vi "Set Properties from Initial.vi"(8 "error in(no error)":errorcluster, 10 "Initial Value":variant, 11 "Properties in":variant) -> (0 "error out":errorcluster, 2 "type":T1, 3 "Properties out":variant)   [LabVIEW 2018, in "Tag Engine.lvlib" / "Tag.lvclass"]
uses:
  Tag.lvclass
  <vilib>/Utility/Data Type/Type Definitions/Data Type.ctl
  <vilib>/Utility/Data Type/NI_Data Type.lvlib
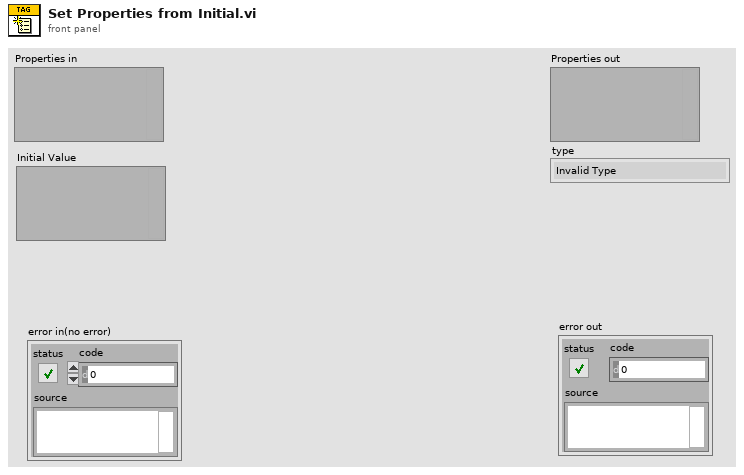
[diagram p1: front panel]
types:
  T1 = typedef "NI_Data Type.lvlib/Data Type.ctl" = enum8{"Invalid Type", "Void", "I8", "I16", "I32", "I64", "U8", "U16", "U32", "U64", "Single Float", "Double Float", "Extended Float", "Single Complex", "Double Complex", "Extended Complex", "Enum U8", "Enum U16", "Enum U32", "Enum U64", "Single Float With Unit", "Double Float With Unit", "Extended Float With Unit", "Single Complex with Unit", "Double Complex with Unit", "Extended Complex with Unit", "Boolean", "String", "Path", "Picture", "Tag", "Array", "Cluster", "Variant", "LV Variant", "Waveform", "Timestamp", "Digital Waveform", "Digital Data", "ExpressData", "Refnum", "External Data", "VI", "Poly VI", "LabVIEW Class Instance", "Fixed Point"}
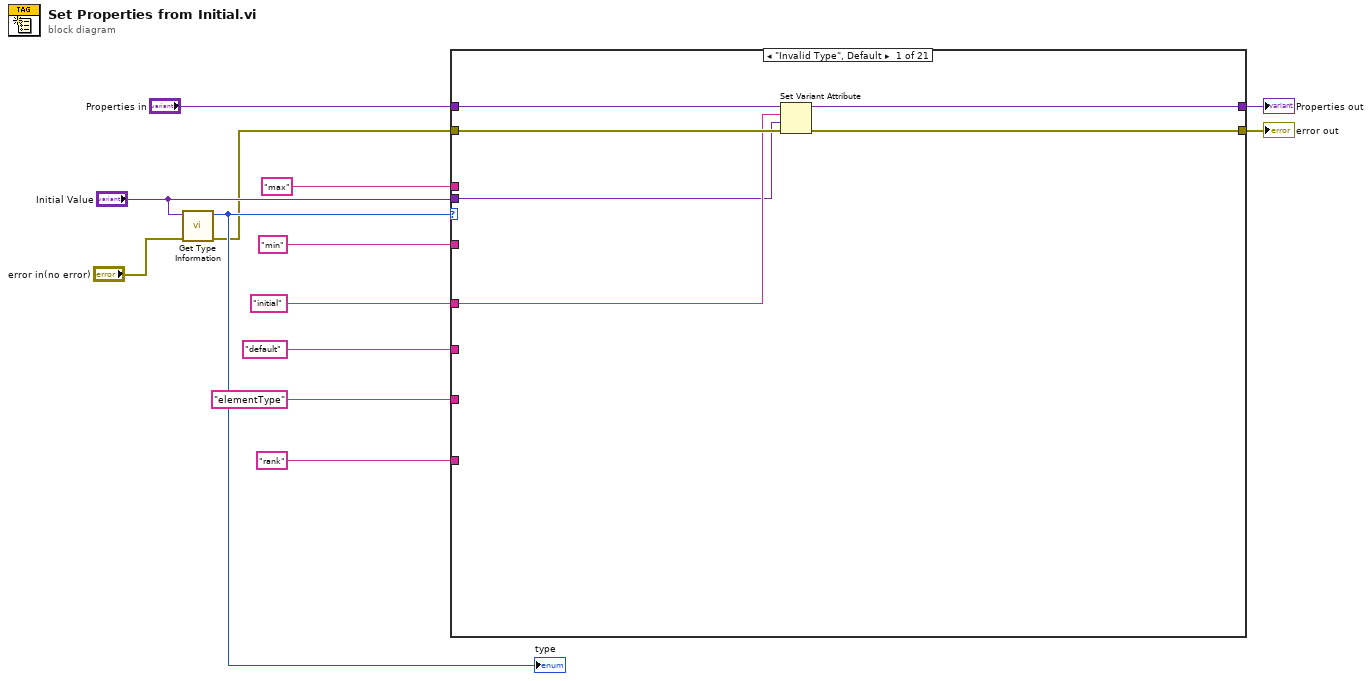
[diagram p0: block diagram]
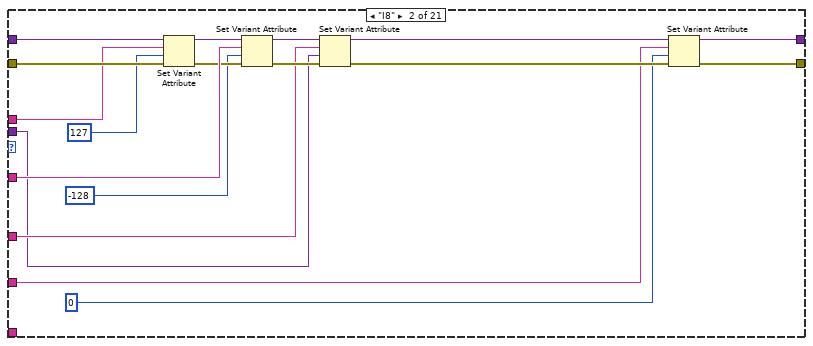
[diagram p2: hidden frame]
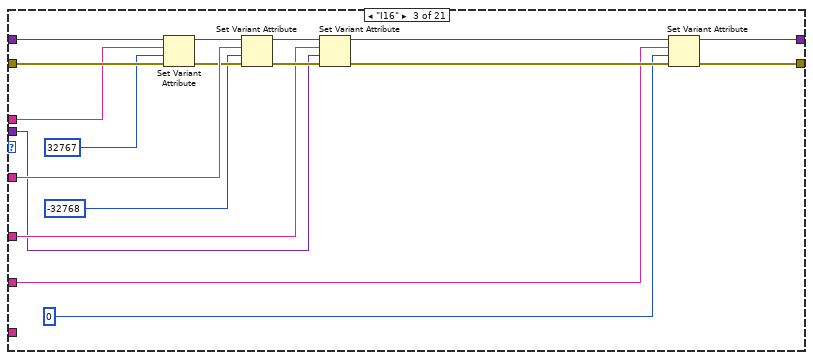
[diagram p3: hidden frame]
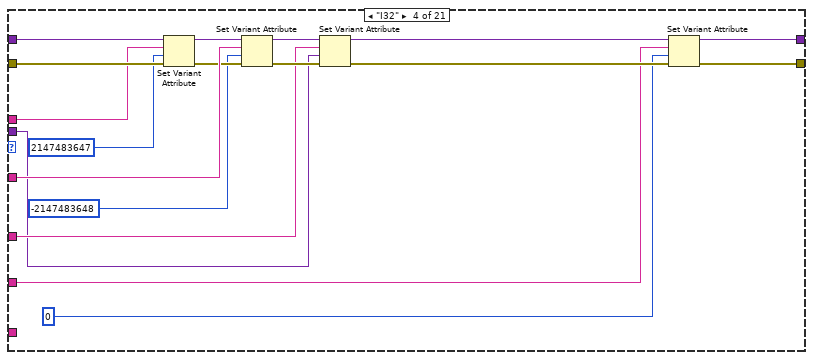
[diagram p4: hidden frame]
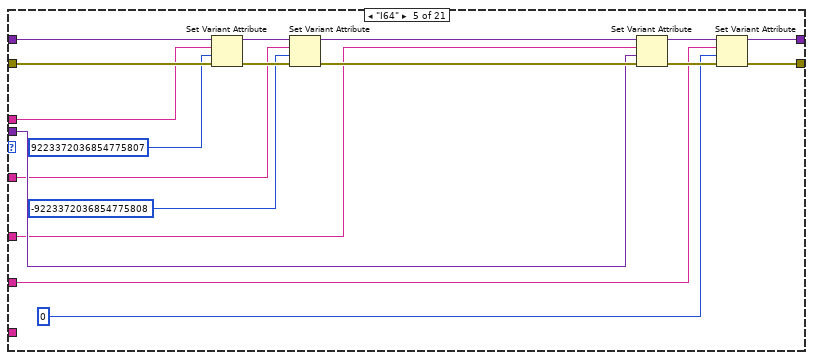
[diagram p5: hidden frame]
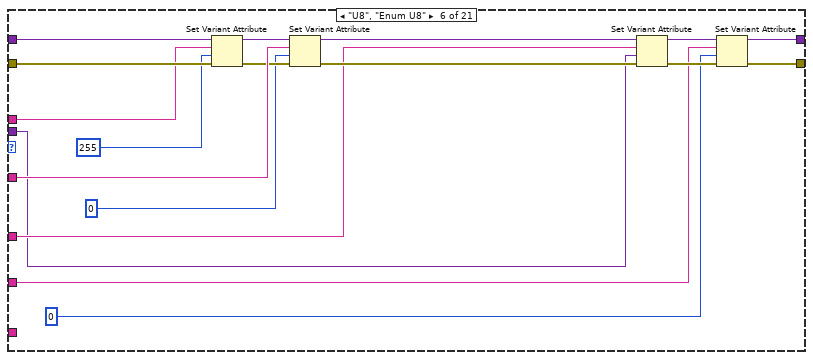
[diagram p6: hidden frame]
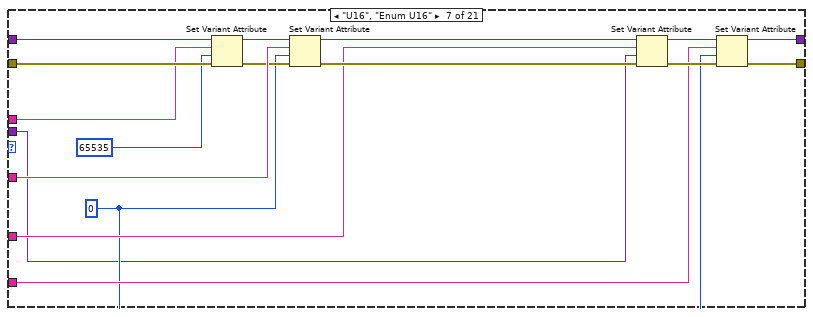
[diagram p7: hidden frame]
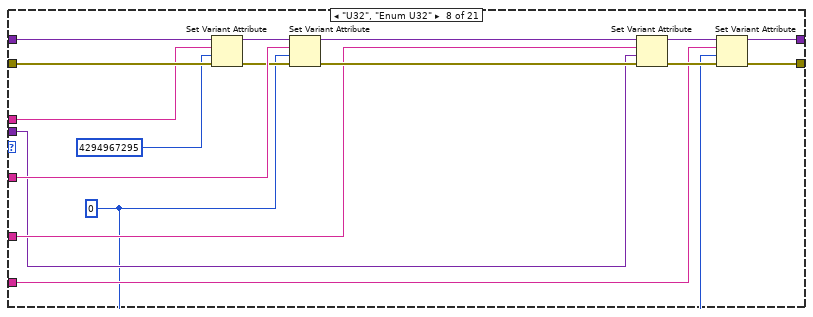
[diagram p8: hidden frame]
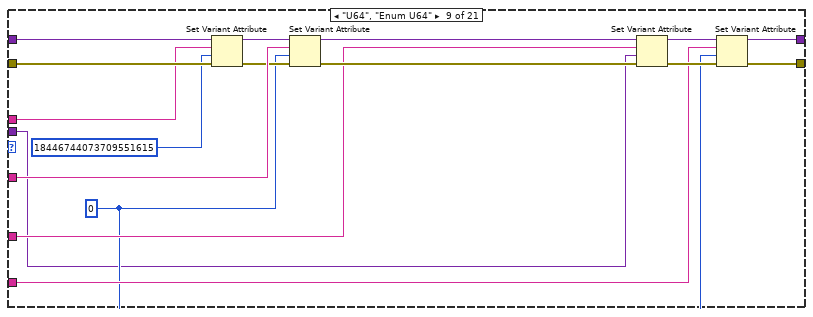
[diagram p9: hidden frame]
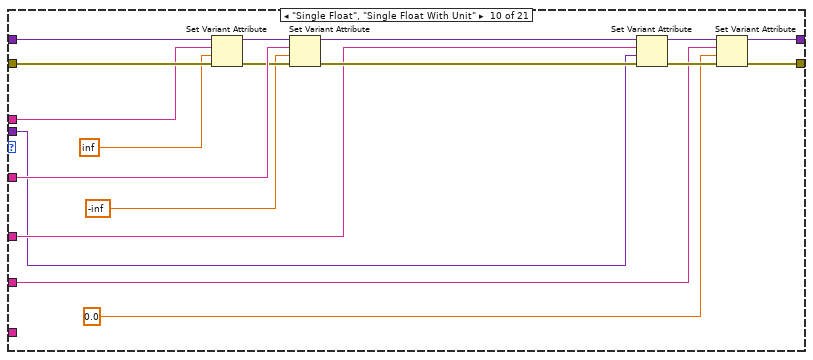
[diagram p10: hidden frame]
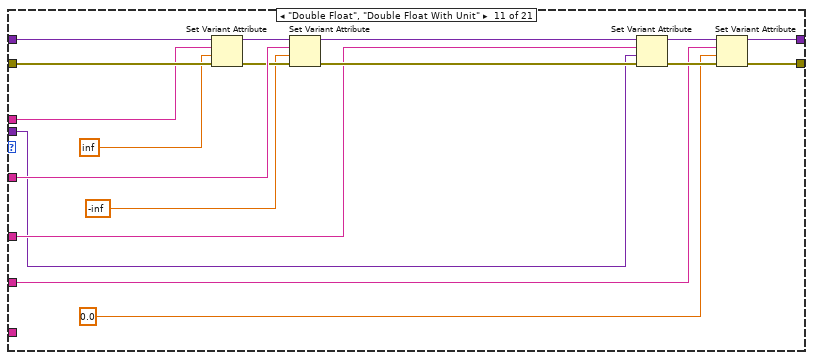
[diagram p11: hidden frame]
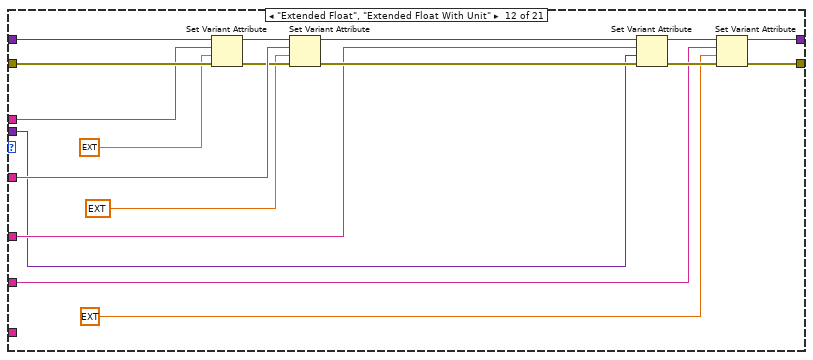
[diagram p12: hidden frame]
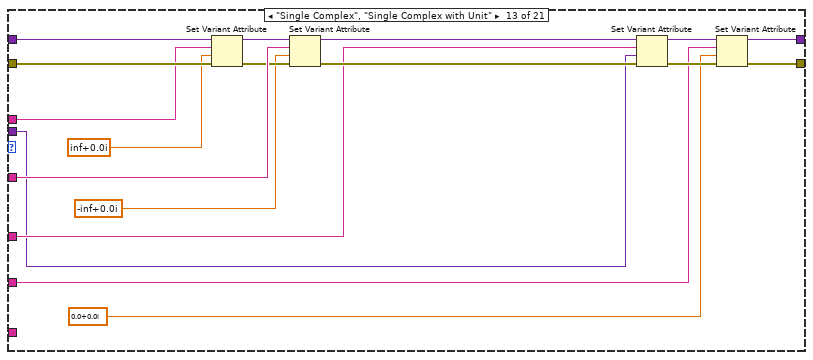
[diagram p13: hidden frame]
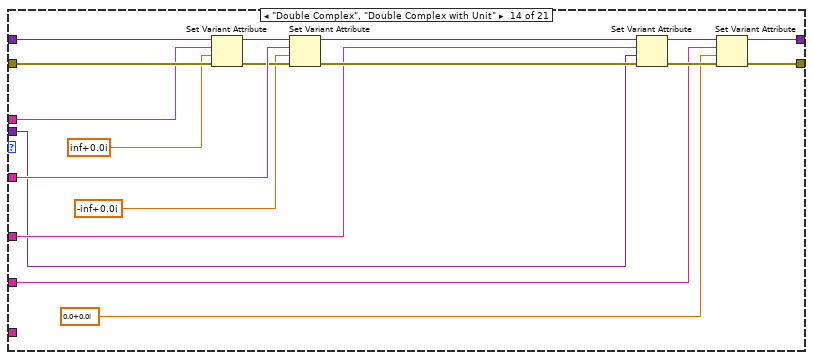
[diagram p14: hidden frame]
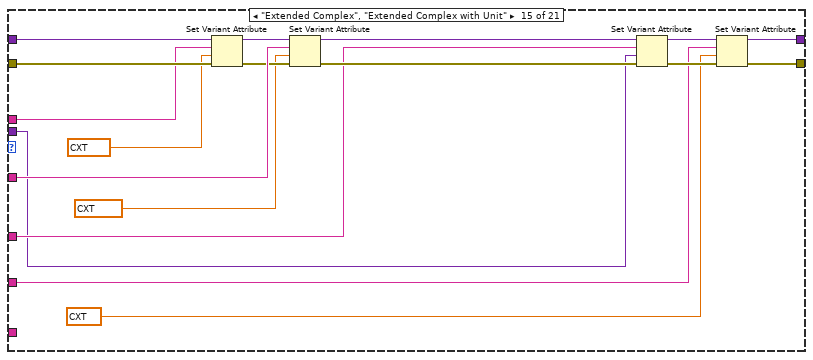
[diagram p15: hidden frame]
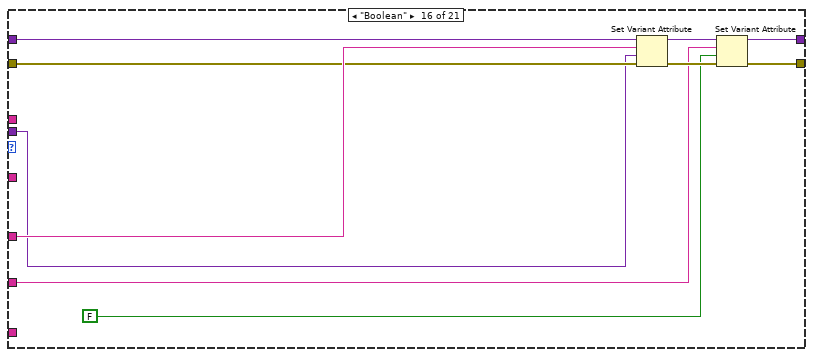
[diagram p16: hidden frame]
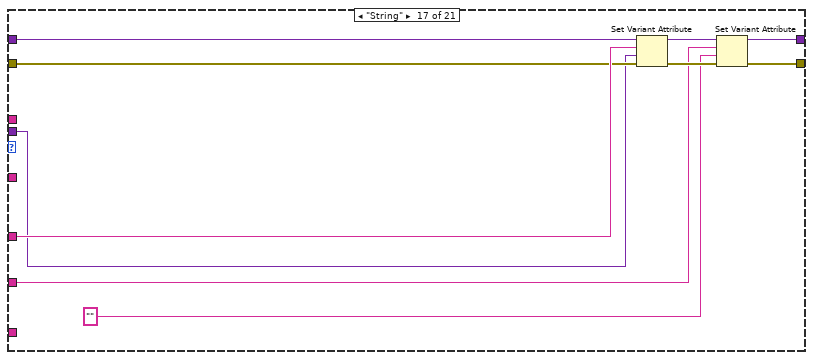
[diagram p17: hidden frame]
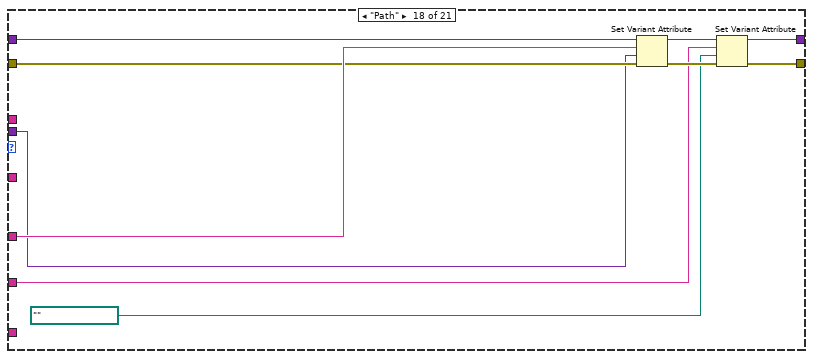
[diagram p18: hidden frame]
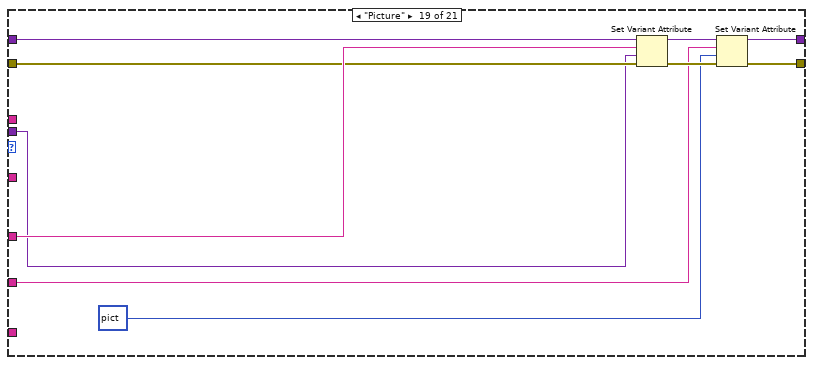
[diagram p19: hidden frame]
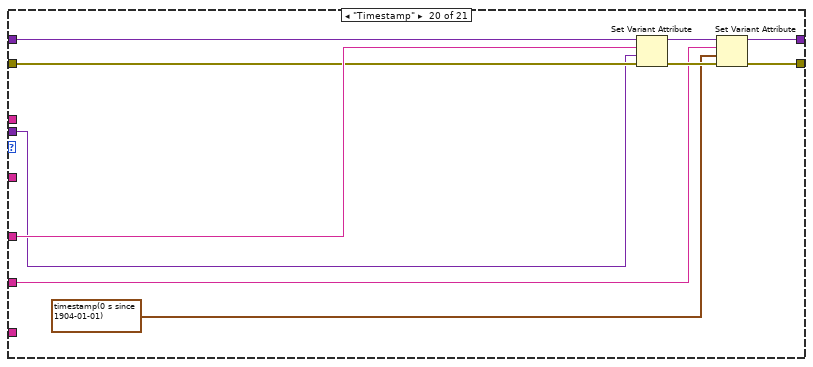
[diagram p20: hidden frame]
diagram:
  n1 = call <vilib>:"Get Type Information.vi"("error in (no error)"="error in(no error)", "Variant"="Initial Value") -> ("error out"=w1:errorcluster, "Type"=w3:T1)  [unwired: 5 in, 3 out]
  "type" <- w3
  n2 = case shown="\"Invalid Type\", Default" w3 {
    tunnel: "Properties in" -> [w19 w37 w55 w73 w91 w109 w126 w143 w160 w178 w196 w214 w232 w250 w268 w272 w282 w292 w302 w312 w327]
    tunnel: "Initial Value" -> [w14 w21 w38 w57 w80 w93 w110 w128 w144 w161 w179 w197 w216 w234 w251 w270 w280 w290 w300 w310 w328]
    tunnel: w1 -> [w18 w36 w54 w72 w90 w108 w125 w142 w159 w177 w195 w213 w231 w249 w267 w271 w281 w291 w301 w311 w326]
    tunnel: "max" ("$Path or Item Name") -> [_ w35 w53 w71 w78 w107 w124 w141 w158 w176 w194 w212 w230 w248 w266 _ _ _ _ _ _]
    tunnel: "min" ("$Path or Item Name") -> [_ w34 w52 w70 w77 w106 w123 w140 w157 w175 w193 w211 w229 w247 w265 _ _ _ _ _ _]
    tunnel: "initial" ("$Path or Item Name") -> [w17 w29 w47 w65 w76 w101 w118 w135 w152 w170 w188 w206 w224 w242 w260 w278 w288 w298 w308 w318 w334]
    tunnel: "default" ("$Path or Item Name") -> [_ w26 w44 w62 w75 w98 w115 w132 w149 w167 w185 w203 w221 w239 w257 w275 w285 w295 w305 w315 _]
    tunnel: [w16 w25 w43 w61 w84 w97 w114 w131 w148 w166 w184 w202 w220 w238 w256 w274 w284 w294 w304 w314 w333] -> w7
    tunnel: [w15 w24 w42 w60 w83 w96 w113 w130 w147 w165 w183 w201 w219 w237 w255 w273 w283 w293 w303 w313 w332] -> w6
    tunnel: "elementType" ("$Path or Item Name") -> [_ _ _ _ _ _ _ _ _ _ _ _ _ _ _ _ _ _ _ _ w322]
    tunnel: "rank" ("$Path or Item Name") -> [_ _ _ _ _ _ _ _ _ _ _ _ _ _ _ _ _ _ _ _ w337]
    frame "Invalid Type", Default {
      n3 = Set Variant Attribute(Variant=w19, name=w17, value=w14, error in=w18) -> (Variant out=w16:variant, error out=w15:errorcluster)  [unwired: 1 out]
    }
    frame "I8" {
      n4 = Set Variant Attribute(Variant=w37, name=w35, value=i8 127, error in=w36) -> (Variant out=w32:variant, error out=w33:errorcluster)  [unwired: 1 out]
      n5 = Set Variant Attribute(Variant=w32, name=w34, value=i8 -128, error in=w33) -> (Variant out=w30:variant, error out=w31:errorcluster)  [unwired: 1 out]
      n6 = Set Variant Attribute(Variant=w30, name=w29, value=w21, error in=w31) -> (Variant out=w28:variant, error out=w27:errorcluster)  [unwired: 1 out]
      n7 = Set Variant Attribute(Variant=w28, name=w26, value=i8 0, error in=w27) -> (Variant out=w25:variant, error out=w24:errorcluster)  [unwired: 1 out]
    }
    frame "I16" {
      n8 = Set Variant Attribute(Variant=w55, name=w53, value=i16 32767, error in=w54) -> (Variant out=w50:variant, error out=w51:errorcluster)  [unwired: 1 out]
      n9 = Set Variant Attribute(Variant=w50, name=w52, value=i16 -32768, error in=w51) -> (Variant out=w48:variant, error out=w49:errorcluster)  [unwired: 1 out]
      n10 = Set Variant Attribute(Variant=w48, name=w47, value=w38, error in=w49) -> (Variant out=w46:variant, error out=w45:errorcluster)  [unwired: 1 out]
      n11 = Set Variant Attribute(Variant=w46, name=w44, value=i16 0, error in=w45) -> (Variant out=w43:variant, error out=w42:errorcluster)  [unwired: 1 out]
    }
    frame "I32" {
      n12 = Set Variant Attribute(Variant=w73, name=w71, value=2147483647, error in=w72) -> (Variant out=w68:variant, error out=w69:errorcluster)  [unwired: 1 out]
      n13 = Set Variant Attribute(Variant=w68, name=w70, value=-2147483648, error in=w69) -> (Variant out=w66:variant, error out=w67:errorcluster)  [unwired: 1 out]
      n14 = Set Variant Attribute(Variant=w66, name=w65, value=w57, error in=w67) -> (Variant out=w64:variant, error out=w63:errorcluster)  [unwired: 1 out]
      n15 = Set Variant Attribute(Variant=w64, name=w62, value=0, error in=w63) -> (Variant out=w61:variant, error out=w60:errorcluster)  [unwired: 1 out]
    }
    frame "I64" {
      n16 = Set Variant Attribute(Variant=w91, name=w78, value=i64 9223372036854775807, error in=w90) -> (Variant out=w88:variant, error out=w89:errorcluster)  [unwired: 1 out]
      n17 = Set Variant Attribute(Variant=w88, name=w77, value=i64 -9223372036854775808, error in=w89) -> (Variant out=w74:variant, error out=w87:errorcluster)  [unwired: 1 out]
      n18 = Set Variant Attribute(Variant=w74, name=w76, value=w80, error in=w87) -> (Variant out=w86:variant, error out=w85:errorcluster)  [unwired: 1 out]
      n19 = Set Variant Attribute(Variant=w86, name=w75, value=i64 0, error in=w85) -> (Variant out=w84:variant, error out=w83:errorcluster)  [unwired: 1 out]
    }
    frame "U8", "Enum U8" {
      n20 = Set Variant Attribute(Variant=w109, name=w107, value=u8 255, error in=w108) -> (Variant out=w104:variant, error out=w105:errorcluster)  [unwired: 1 out]
      n21 = Set Variant Attribute(Variant=w104, name=w106, value=u8 0, error in=w105) -> (Variant out=w102:variant, error out=w103:errorcluster)  [unwired: 1 out]
      n22 = Set Variant Attribute(Variant=w102, name=w101, value=w93, error in=w103) -> (Variant out=w100:variant, error out=w99:errorcluster)  [unwired: 1 out]
      n23 = Set Variant Attribute(Variant=w100, name=w98, value=u8 0, error in=w99) -> (Variant out=w97:variant, error out=w96:errorcluster)  [unwired: 1 out]
    }
    frame "U16", "Enum U16" {
      w111 = u16 0
      n24 = Set Variant Attribute(Variant=w126, name=w124, value=u16 65535, error in=w125) -> (Variant out=w121:variant, error out=w122:errorcluster)  [unwired: 1 out]
      n25 = Set Variant Attribute(Variant=w121, name=w123, value=w111, error in=w122) -> (Variant out=w119:variant, error out=w120:errorcluster)  [unwired: 1 out]
      n26 = Set Variant Attribute(Variant=w119, name=w118, value=w110, error in=w120) -> (Variant out=w117:variant, error out=w116:errorcluster)  [unwired: 1 out]
      n27 = Set Variant Attribute(Variant=w117, name=w115, value=w111, error in=w116) -> (Variant out=w114:variant, error out=w113:errorcluster)  [unwired: 1 out]
    }
    frame "U32", "Enum U32" {
      w127 = u32 0
      n28 = Set Variant Attribute(Variant=w143, name=w141, value=u32 4294967295, error in=w142) -> (Variant out=w138:variant, error out=w139:errorcluster)  [unwired: 1 out]
      n29 = Set Variant Attribute(Variant=w138, name=w140, value=w127, error in=w139) -> (Variant out=w136:variant, error out=w137:errorcluster)  [unwired: 1 out]
      n30 = Set Variant Attribute(Variant=w136, name=w135, value=w128, error in=w137) -> (Variant out=w134:variant, error out=w133:errorcluster)  [unwired: 1 out]
      n31 = Set Variant Attribute(Variant=w134, name=w132, value=w127, error in=w133) -> (Variant out=w131:variant, error out=w130:errorcluster)  [unwired: 1 out]
    }
    frame "U64", "Enum U64" {
      w145 = u64 0
      n32 = Set Variant Attribute(Variant=w160, name=w158, value=u64 18446744073709551615, error in=w159) -> (Variant out=w155:variant, error out=w156:errorcluster)  [unwired: 1 out]
      n33 = Set Variant Attribute(Variant=w155, name=w157, value=w145, error in=w156) -> (Variant out=w153:variant, error out=w154:errorcluster)  [unwired: 1 out]
      n34 = Set Variant Attribute(Variant=w153, name=w152, value=w144, error in=w154) -> (Variant out=w151:variant, error out=w150:errorcluster)  [unwired: 1 out]
      n35 = Set Variant Attribute(Variant=w151, name=w149, value=w145, error in=w150) -> (Variant out=w148:variant, error out=w147:errorcluster)  [unwired: 1 out]
    }
    frame "Single Float", "Single Float With Unit" {
      n36 = Set Variant Attribute(Variant=w178, name=w176, value=sgl inf, error in=w177) -> (Variant out=w173:variant, error out=w174:errorcluster)  [unwired: 1 out]
      n37 = Set Variant Attribute(Variant=w173, name=w175, value=sgl -inf, error in=w174) -> (Variant out=w171:variant, error out=w172:errorcluster)  [unwired: 1 out]
      n38 = Set Variant Attribute(Variant=w171, name=w170, value=w161, error in=w172) -> (Variant out=w169:variant, error out=w168:errorcluster)  [unwired: 1 out]
      n39 = Set Variant Attribute(Variant=w169, name=w167, value=sgl 0.0, error in=w168) -> (Variant out=w166:variant, error out=w165:errorcluster)  [unwired: 1 out]
    }
    frame "Double Float", "Double Float With Unit" {
      n40 = Set Variant Attribute(Variant=w196, name=w194, value=inf, error in=w195) -> (Variant out=w191:variant, error out=w192:errorcluster)  [unwired: 1 out]
      n41 = Set Variant Attribute(Variant=w191, name=w193, value=-inf, error in=w192) -> (Variant out=w189:variant, error out=w190:errorcluster)  [unwired: 1 out]
      n42 = Set Variant Attribute(Variant=w189, name=w188, value=w179, error in=w190) -> (Variant out=w187:variant, error out=w186:errorcluster)  [unwired: 1 out]
      n43 = Set Variant Attribute(Variant=w187, name=w185, value=0.0, error in=w186) -> (Variant out=w184:variant, error out=w183:errorcluster)  [unwired: 1 out]
    }
    frame "Extended Float", "Extended Float With Unit" {
      n44 = Set Variant Attribute(Variant=w214, name=w212, value=ext inf, error in=w213) -> (Variant out=w209:variant, error out=w210:errorcluster)  [unwired: 1 out]
      n45 = Set Variant Attribute(Variant=w209, name=w211, value=ext -inf, error in=w210) -> (Variant out=w207:variant, error out=w208:errorcluster)  [unwired: 1 out]
      n46 = Set Variant Attribute(Variant=w207, name=w206, value=w197, error in=w208) -> (Variant out=w205:variant, error out=w204:errorcluster)  [unwired: 1 out]
      n47 = Set Variant Attribute(Variant=w205, name=w203, value=ext 0.0, error in=w204) -> (Variant out=w202:variant, error out=w201:errorcluster)  [unwired: 1 out]
    }
    frame "Single Complex", "Single Complex with Unit" {
      n48 = Set Variant Attribute(Variant=w232, name=w230, value=csg inf+0.0i, error in=w231) -> (Variant out=w227:variant, error out=w228:errorcluster)  [unwired: 1 out]
      n49 = Set Variant Attribute(Variant=w227, name=w229, value=csg -inf+0.0i, error in=w228) -> (Variant out=w225:variant, error out=w226:errorcluster)  [unwired: 1 out]
      n50 = Set Variant Attribute(Variant=w225, name=w224, value=w216, error in=w226) -> (Variant out=w223:variant, error out=w222:errorcluster)  [unwired: 1 out]
      n51 = Set Variant Attribute(Variant=w223, name=w221, value=csg 0.0+0.0i, error in=w222) -> (Variant out=w220:variant, error out=w219:errorcluster)  [unwired: 1 out]
    }
    frame "Double Complex", "Double Complex with Unit" {
      n52 = Set Variant Attribute(Variant=w250, name=w248, value=cdb inf+0.0i, error in=w249) -> (Variant out=w245:variant, error out=w246:errorcluster)  [unwired: 1 out]
      n53 = Set Variant Attribute(Variant=w245, name=w247, value=cdb -inf+0.0i, error in=w246) -> (Variant out=w243:variant, error out=w244:errorcluster)  [unwired: 1 out]
      n54 = Set Variant Attribute(Variant=w243, name=w242, value=w234, error in=w244) -> (Variant out=w241:variant, error out=w240:errorcluster)  [unwired: 1 out]
      n55 = Set Variant Attribute(Variant=w241, name=w239, value=cdb 0.0+0.0i, error in=w240) -> (Variant out=w238:variant, error out=w237:errorcluster)  [unwired: 1 out]
    }
    frame "Extended Complex", "Extended Complex with Unit" {
      n56 = Set Variant Attribute(Variant=w268, name=w266, value=cxt inf+0.0i, error in=w267) -> (Variant out=w263:variant, error out=w264:errorcluster)  [unwired: 1 out]
      n57 = Set Variant Attribute(Variant=w263, name=w265, value=cxt -inf+0.0i, error in=w264) -> (Variant out=w261:variant, error out=w262:errorcluster)  [unwired: 1 out]
      n58 = Set Variant Attribute(Variant=w261, name=w260, value=w251, error in=w262) -> (Variant out=w259:variant, error out=w258:errorcluster)  [unwired: 1 out]
      n59 = Set Variant Attribute(Variant=w259, name=w257, value=cxt 0.0+0.0i, error in=w258) -> (Variant out=w256:variant, error out=w255:errorcluster)  [unwired: 1 out]
    }
    frame "Boolean" {
      n60 = Set Variant Attribute(Variant=w272, name=w278, value=w270, error in=w271) -> (Variant out=w277:variant, error out=w276:errorcluster)  [unwired: 1 out]
      n61 = Set Variant Attribute(Variant=w277, name=w275, value=FALSE, error in=w276) -> (Variant out=w274:variant, error out=w273:errorcluster)  [unwired: 1 out]
    }
    frame "String" {
      n62 = Set Variant Attribute(Variant=w282, name=w288, value=w280, error in=w281) -> (Variant out=w287:variant, error out=w286:errorcluster)  [unwired: 1 out]
      n63 = Set Variant Attribute(Variant=w287, name=w285, value="", error in=w286) -> (Variant out=w284:variant, error out=w283:errorcluster)  [unwired: 1 out]
    }
    frame "Path" {
      n64 = Set Variant Attribute(Variant=w292, name=w298, value=w290, error in=w291) -> (Variant out=w297:variant, error out=w296:errorcluster)  [unwired: 1 out]
      n65 = Set Variant Attribute(Variant=w297, name=w295, value=path "", error in=w296) -> (Variant out=w294:variant, error out=w293:errorcluster)  [unwired: 1 out]
    }
    frame "Picture" {
      n66 = Set Variant Attribute(Variant=w302, name=w308, value=w300, error in=w301) -> (Variant out=w307:variant, error out=w306:errorcluster)  [unwired: 1 out]
      n67 = Set Variant Attribute(Variant=w307, name=w305, value=picture data[5B] ("empty picture"), error in=w306) -> (Variant out=w304:variant, error out=w303:errorcluster)  [unwired: 1 out]
    }
    frame "Timestamp" {
      n68 = Set Variant Attribute(Variant=w312, name=w318, value=w310, error in=w311) -> (Variant out=w317:variant, error out=w316:errorcluster)  [unwired: 1 out]
      n69 = Set Variant Attribute(Variant=w317, name=w315, value=timestamp(0 s since 1904-01-01), error in=w316) -> (Variant out=w314:variant, error out=w313:errorcluster)  [unwired: 1 out]
    }
    frame "Array" {
      # "Set Max,Min,Default"
      n70 = call <vilib>:"Get Array Information.vi"("error in (no error)"=w326, "Variant"=w328) -> ("error out"=w321:errorcluster, "Array Element Data Type"=w329:variant, "Number of Dimensions"=w331:i32)  [unwired: 6 in, 1 out]
      n71 = To Unsigned Byte Integer(number=w331) -> (unsigned 8bit integer=w330:u8)
      n72 = Set Variant Attribute(Variant=w327, name=w337, value=w330, error in=w321) -> (Variant out=w336:variant, error out=w335:errorcluster)  [unwired: 1 out]
      n73 = call "Set Properties from Initial.vi"("error in(no error)"=w335, "Initial Value"=w329, "Properties in"=w336) -> ("error out"=w324:errorcluster, "type"=w323:T1, "Properties out"=w325:variant)  [unwired: 6 in]
      n74 = Set Variant Attribute(Variant=w325, name=w322, value=w323, error in=w324) -> (Variant out=w319:variant, error out=w320:errorcluster)  [unwired: 1 out]
      n75 = Set Variant Attribute(Variant=w319, name=w334, value=w328, error in=w320) -> (Variant out=w333:variant, error out=w332:errorcluster)  [unwired: 1 out]
    }
  }
  "Properties out" <- w7
  "error out" <- w6
